vi "Test Multiply.vi"() -> ()   [LabVIEW 2014]
uses:
  Complex Numbers.lvlib
panel:
  out "Divide":u32
  out "Error Out":errorcluster
  in  "Error In":errorcluster
  out "Multiply":u32
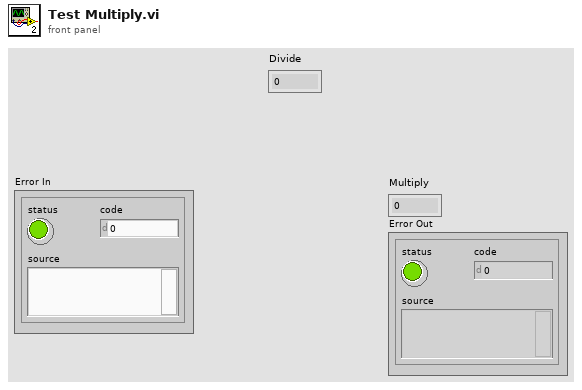
[diagram p1: front panel]
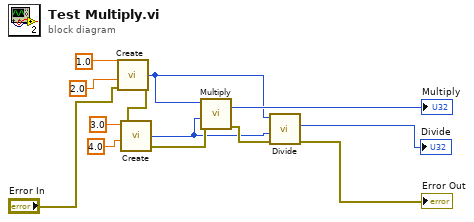
[diagram p0: block diagram]
diagram:
  n1 = call "Create.vi"("Error In"="Error In", "Imag"=2.0 ("Real"), "Real"=1.0) -> ("Error Out"=w10:errorcluster, "Complex"=w3:u32)  [unwired: 2 in]
  n2 = call "Create.vi"("Error In"=w10, "Imag"=4.0 ("Real"), "Real"=3.0) -> ("Error Out"=w7:errorcluster, "Complex"=w4:u32)  [unwired: 2 in]
  n3 = call "Multiply.vi"("Error In"=w7, "B"=w4, "A"=w3) -> ("Error Out"=w5:errorcluster, "result"=→"Multiply":u32)  [unwired: 7 in]
  n4 = call "Divide.vi"("Error In"=w5, "B"=w4, "A"=w3) -> ("Error Out"=→"Error Out":errorcluster, "result"=→"Divide":u32)  [unwired: 7 in]
